vi "nominal_channel_writer.write_batches.from_waveform.request.vi"(8 "error in":errorcluster, 9 "Waveform":waveform(dbl), 10 "Channel":string, 11 "Data Source RID":string) -> (0 "error out":errorcluster, 3 "Response body":string)   [LabVIEW 2020, in "Nominal Client.lvclass"]
doc: "Synchronously writes batches of records to a Nominal data source.\n\nTAGS:\nThis is a malleable VI (VIM) that will accept:\n- Map: Name (String) -> Value (String)\n- Array of Clusters: {Name (String), Value (String)}\n- Cluster: {Array of Names (String), Array of Values (String)}"
uses:
  Nominal Client.lvclass
  21b7f8af-3caf-483d-a354-f1bbe3edb404.vi
  2c8a2fb0-06af-4bda-9dcc-d72a85547e70.vi
  028fdd67-09da-40c6-8995-0c4bd62a0b31.vi
  c2a1aca9-ea5a-4b2a-8072-18de54756c53.vi
  <vilib>/LabVIEW Open Source Project/Epoch Date & Time/epoch.UNIX/Epoch.UNIX.lvclass
  C:/Program Files/National Instruments/LabVIEW 2020/vi.lib/LabVIEW Open Source Project/Epoch Date & Time/epoch/Epoch.lvclass
  <vilib>/LabVIEW Open Source Project/Epoch Date & Time/Get Epoch Time.vi
  <vilib>/JDP Science/JSONtext/Variant to JSON Text.vi
  <vilib>/JDP Science/JSONtext/support/Format JSON Object.vi
  <vilib>/JDP Science/JSONtext/LVClass Serializer/JSONtext LVClass Serializer.lvclass
  Nominal Client.lvclass/Nominal Client.ctl
  <vilib>/JDP Science/JSONtext/JSONtext.lvlib
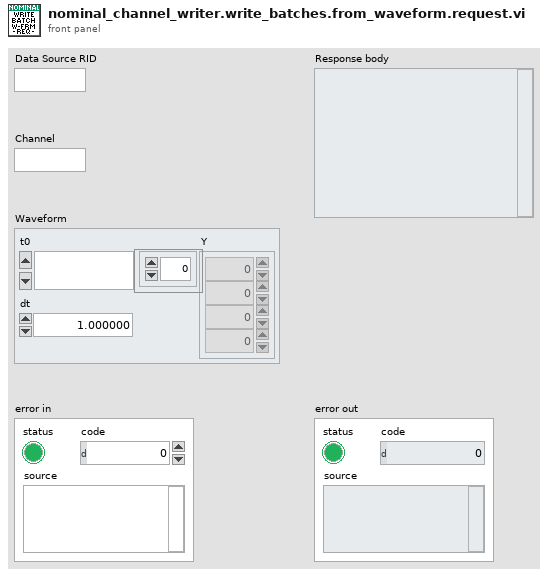
[diagram p1: front panel]
types:
  T1 = cluster{"type":string, "double":cluster{"timestamp":cluster{"seconds":i32, "nanos":i32}, "value":dbl}[]}
  T2 = cluster{"UNIX Timestamp":cluster{"Seconds":i64, "Nanoseconds":i64}, dbl}
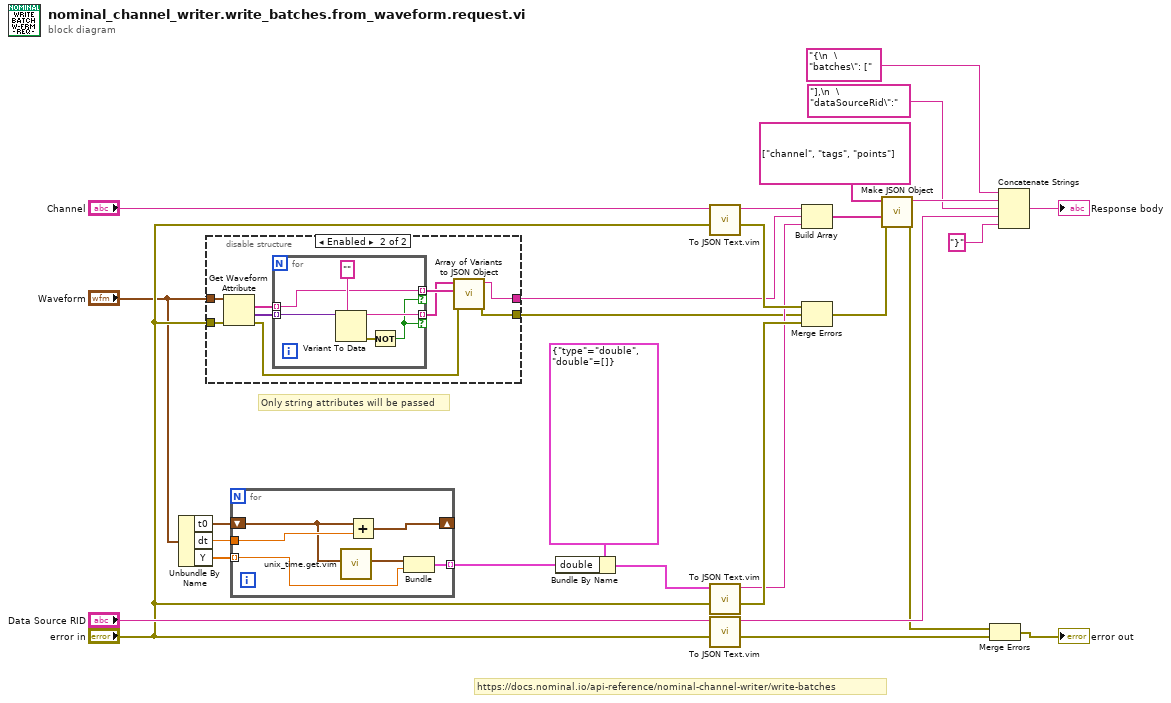
[diagram p0: block diagram]
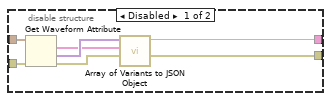
[diagram p2: hidden frame]
diagram:
  # "Only string attributes will be passed"
  # "https://docs.nominal.io/api-reference/nominal-channel-writer/write-batches"
  n1 = Unbundle By Name("Waveform") -> ("t0"=w24:timestamp, "dt"=w23:dbl, "Y"=w25:dbl[])
  n2 = disable-structure shown="Enabled" {
    disable-tunnel: "error in" -> [w35 w44]
    disable-tunnel: "Waveform" -> [w34 w43]
    disable-tunnel: [w30 w38] -> w11
    disable-tunnel: [w29 w37] -> w10
    frame Disabled {
      n3 = Get Waveform Attribute(4:w35, 7:w34) -> (0:w31:errorcluster, 1:w33:variant[], 2:w32:string[])  [unwired: 2 in, 1 out]
      n4 = call <vilib>:"Array of Variants to JSON Object.vi"("error in (no error)"=w31, "Names"=w32, "Array"=w33) -> ("error out"=w29:errorcluster, "<JSON>"=w30:string)  [unwired: 7 in]
    }
    frame Enabled {
      n5 = Get Waveform Attribute(4:w44, 7:w43) -> (0:w36:errorcluster, 1:w42:variant[], 2:w41:string[])  [unwired: 2 in, 1 out]
      n6 = for {
        tunnel: w42 -> [w50] mode=indexing
        tunnel: w41 -> [w46] mode=indexing
        tunnel: [w48] -> w39 mode=indexing if=w45
        tunnel: [w46] -> w40 mode=indexing if=w45
        n7 = Variant To Data(type="", Variant=w50) -> (data=w48:string, error out=w47:errorcluster)  [unwired: 1 in]
        n8 = Not(x=w47) -> (.not. x?=w45:bool)
      }
      n9 = call <vilib>:"Array of Variants to JSON Object.vi"("error in (no error)"=w36, "Names"=w40, "Array"=w39) -> ("error out"=w37:errorcluster, "<JSON>"=w38:string)  [unwired: 7 in]
    }
  }
  n10 = for {
    tunnel: w25 -> [w52] mode=indexing
    tunnel: w23 -> [w56]
    shift-right: [w55] -> _
    shift-left: w24 -> [w54]
    tunnel: [w51] -> w21 mode=indexing
    n11 = call "unix_time.get.vim"("Time Stamp (empty: now) [single or array]"=w54) -> ("UNIX Timestamp"=w53:cluster{"Seconds":i64, "Nanoseconds":i64})  [unwired: 10 in]
    n12 = Add(x=w54, y=w56) -> (x+y=w55:timestamp)
    n13 = Bundle("UNIX Timestamp"=w53, w52) -> (w51:T2)  [unwired: 1 in]
  }
  n14 = Bundle By Name(cluster=T1 {"type"="double", "double"=[]}, "double"=w21) -> (w20:T1)
  n15 = call "To JSON Text.vim"("error in (no error)"="error in", "Anything"="Channel") -> ("error out"=w27:errorcluster, "<JSON>"=w18:string)  [unwired: 8 in]
  n16 = call "To JSON Text.vim"("error in (no error)"="error in", "Anything"=w20) -> ("error out"=w28:errorcluster, "<JSON>"=w19:string)  [unwired: 8 in]
  n17 = call "To JSON Text.vim"("error in (no error)"="error in", "Anything"="Data Source RID") -> ("error out"=w2:errorcluster, "<JSON>"=w5:string)  [unwired: 8 in]
  n18 = Build Array(w18, w11, w19) -> (w17:string[])
  n19 = Merge Errors(w27, w10, w28) -> (w15:errorcluster)
  n20 = call <vilib>:"Make JSON Object.vi"("error in (no error)"=w15, "JSON Items"=w17, "Item Names"=string[] ["channel", "tags", "points"]) -> ("error out"=w3:errorcluster, "<JSON>"=w9:string)  [unwired: 7 in]
  n21 = Merge Errors(w3, w2) -> (→"error out":errorcluster)
  n22 = Concatenate Strings("{\n  \"batches\": [" ("string"), w9, "],\n  \"dataSourceRid\":" ("string"), w5, "}" ("string")) -> (→"Response body":string)
